vi "DpcPutReg.vi"(8 "Error In":errorcluster, 9 "Data":u8, 10 "Register Address":u8, 11 "Device Handle":u32) -> (0 "Error Out":errorcluster, 2 "Task ID":u16, 3 "Device Hanle":u32)   [LabVIEW 2011, in "LVH-Adept.lvlib" / "DPCUTIL.lvlib"]
uses:
  DPCUTIL.lvlib
  Private/Type Defs/Error.ctl
  Resources/dpcutil.dll
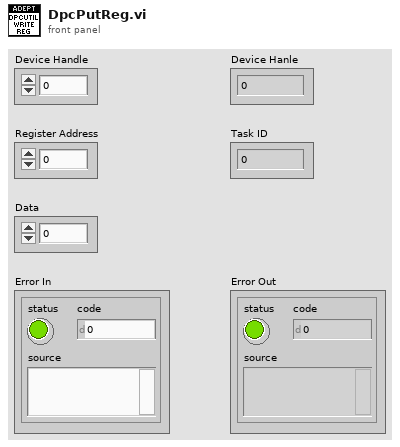
[diagram p1: front panel]
types:
  T1 = typedef "LVH-Adept.lvlib/DPCUTIL.lvlib/Error.ctl" = enum16{"Unknown", "Open Data", "Wait For Transaction", "Put Reg", "Get Reg", "Close Data"}
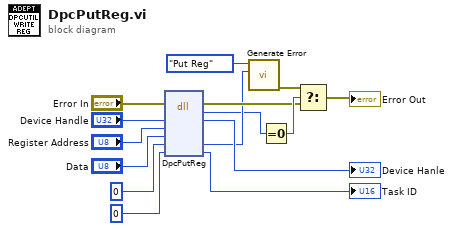
[diagram p0: block diagram]
diagram:
  n1 = dll-call lib="C:/github/labviewhacker/LVH-Adept/LabVIEW/vi.lib/LabVIEW Hacker/Adept/Private/Resources/dpcutil.*" fn="DpcPutReg"(error in="Error In", "hif"="Device Handle", "bAddr"="Register Address", "bData"="Data", "perc"=0, "ptrid"=u16 0) -> (error out=w3:errorcluster, w1:i32, "hif"=→"Device Hanle":u32, "perc"=w2:i32, "ptrid"=→"Task ID":u16)  [unwired: 4 in, 1 out]
  n2 = call "Generate Error.vi"("Adept Error Code"=w2, "DPCUTIL Error"=Error."Put Reg") -> ("Error Out"=w7:errorcluster)  [unwired: 9 in]
  n3 = Equal To 0?(x=w1) -> (x = 0?=w6:bool)
  n4 = Select(t=w7, s=w6, f=w3) -> (s? t:f=→"Error Out":errorcluster)
